vi "Stop Core.vi"(10 "final error code":i32, 11 "ServerListener in":refnum<class "ServerListener.lvclass">) -> (3 "ServerListener out":refnum<class "ServerListener.lvclass">)   [LabVIEW 2016, in "ServerListener.lvlib" / "ServerListener.lvclass"]
doc: "(<B>Filename</B>: Actor Framework.lvlib:Actor.lvclass:Stop Core.vi)\n\nDefines what the actor does before it stops. Use the <B>final error code</B> input to determine whether the actor shut down in response to an error.\n\nBy default, this method does nothing. A descendant class may override it to define behavior, such as shutting down any processes the actor initiated in its override of the Actor Core method."
uses:
  ServerListener.lvclass
  C:/Program Files (x86)/National Instruments/LabVIEW 2016/vi.lib/ActorFramework/Actor/Actor.lvclass
  ServerListener.lvclass/ServerListener.ctl
  <vilib>/ActorFramework/Actor/Actor.lvclass/Actor.ctl
  <vilib>/ActorFramework/Message Enqueuer/Message Enqueuer.lvclass/Message Enqueuer.ctl
  <vilib>/ActorFramework/Message Enqueuer/Enqueue.vi
  Controller/Messages/Server Listener Stopped Msg/Server Listener Stopped Msg.lvclass
  C:/Program Files (x86)/National Instruments/LabVIEW 2016/vi.lib/ActorFramework/Message/Message.lvclass
  <vilib>/ActorFramework/Message Priority Queue/Priority Enqueue.vi
  <vilib>/ActorFramework/Actor/Actor.lvclass
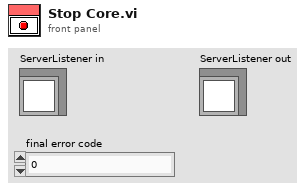
[diagram p1: front panel]
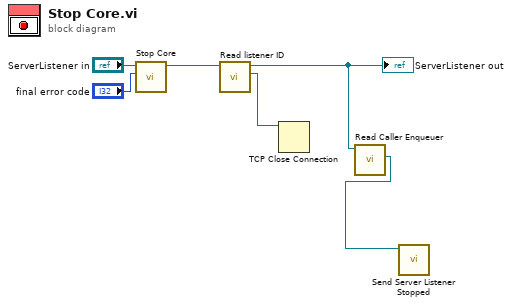
[diagram p0: block diagram]
diagram:
  n1 = call-parent "Stop Core.vi"("final error code"="final error code", "Actor in"="ServerListener in") -> ("Actor out"=w4:refnum<class "ServerListener.lvclass">)  [unwired: 9 in]
  n2 = call "Read listener ID.vi"("ServerListener in"=w4) -> ("listener ID"=w3:refnum<k5>, "ServerListener out"=w2:refnum<class "ServerListener.lvclass">)  [unwired: 8 in, 1 out]
  "ServerListener out" <- w2
  n3 = TCP Close Connection(connection ID=w3) -> ()  [unwired: 2 in, 2 out]
  n4 = call <vilib>:"Read Caller Enqueuer.vi"("Actor"=w2) -> ("Caller Enqueuer"=w1:refnum<class "Message Enqueuer.lvclass">)  [unwired: 10 in]
  n5 = call "Send Server Listener Stopped.vi"("Message Enqueuer"=w1) -> ()  [unwired: 9 in, 2 out]
